vi "GetSecondsInBlock.vi"(8 "error in (no error)":errorcluster, 9 "desired length":dbl, 10 "block in":T1, 11 "data group":string) -> (0 "error out":errorcluster, 1 "total seconds":dbl, 2 "complete":bool, 3 "index of last":i32, 5 "extra seconds":dbl)   [LabVIEW 2017, in "DVRBuffer.lvlib"]
uses:
  <vilib>/addons/InsightCM/Devices/Shared/Common/DVRBuffer/DVRBuffer.lvlib
  <vilib>/addons/InsightCM/Devices/Shared/Common/DVRBuffer/controls/BufferLocation.ctl
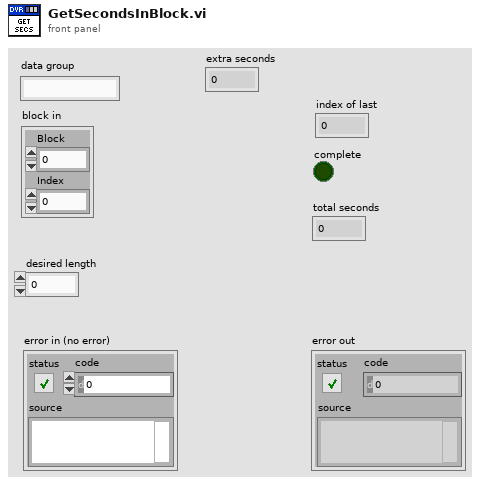
[diagram p1: front panel]
types:
  T1 = typedef "DVRBuffer.lvlib/BufferLocation.ctl" = cluster{"Block":u32, "Index":i32}
  T2 = typedef "DVRBuffer.lvlib/DVRElement.ctl" = cluster{"location":u32, "DVR":u32, "points":i32, "dt":dbl, "PulsePositions":dbl[], "Pulses Per Rev":dbl}
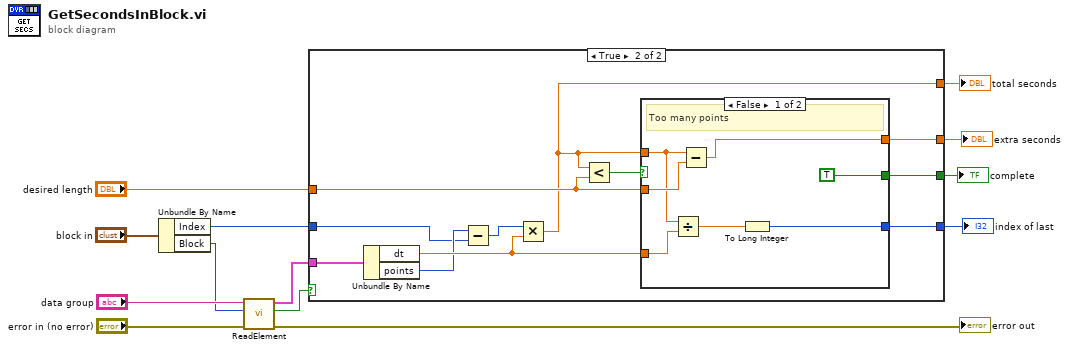
[diagram p0: block diagram]
diagram:
  n1 = Unbundle By Name("block in") -> ("Index"=w9:i32, "Block"=w2:u32)
  n2 = call <vilib>:"ReadElement.vi"("error in (no error)"="error in (no error)", "buffer location"=w2, "name"="data group") -> ("error out"=→"error out":errorcluster, "found"=w3:bool, "DVR element"=w8:T2)  [unwired: 6 in]
  n3 = case shown="True" w3 {
    tunnel: w9 -> [w14 w17]
    tunnel: "desired length" -> [_ w23]
    tunnel: w8 -> [_ w25]
    tunnel: [w14 w18] -> w7
    tunnel: [_ w19] -> w4
    tunnel: [_ w16] -> w6
    tunnel: [_ w15] -> w1
    frame False {
    }
    frame True {
      n4 = Unbundle By Name(w25) -> ("dt"=w22:dbl, "points"=w21:i32)
      n5 = Subtract(x=w21, y=w17) -> (x-y=w20:i32)
      n6 = Multiply(x=w20, y=w22) -> (x*y=w16:dbl)
      n7 = Less?(x=w16, y=w23) -> (x < y?=w24:bool)
      n8 = case shown="False" w24 {
        tunnel: w16 -> [w26 _]
        tunnel: w23 -> [w32 _]
        tunnel: w22 -> [w31 _]
        tunnel: [w28 _] -> w18
        tunnel: [TRUE _] -> w19
        tunnel: [w27 _] -> w15
        frame False {
          # "Too many points"
          n9 = Divide(x=w26, y=w31) -> (x/y=w30:dbl)
          n10 = Subtract(x=w26, y=w32) -> (x-y=w27:dbl)
          n11 = To Long Integer(number=w30) -> (32bit integer=w28:i32)
        }
        frame True {
          # "Not enough points"
        }
      }
    }
  }
  "total seconds" <- w6
  "complete" <- w4
  "index of last" <- w7
  "extra seconds" <- w1
